vi "TestingPoint.vi"() -> ()   [LabVIEW 2016]
uses:
  <vilib>/Rock Robotics/WPI/Utilities/WPI_GetSetVariantRefNum.vi
panel:
  in  "Zero Yaw":bool
  in  "Config":T1={"Angle"=360.0, "MaxVelocity"=60.0, "MaxAccel"=50.0, "InitialVelocity"=0.0, "FinalVelocity"=0.0}
  out "Outputs":dbl(graph)
  in  "Go":bool
  in  "Go Backwards":bool
  out "Angular velocity":cluster{dbl, "vel":dbl}(graph)
  out "Angle":cluster{dbl, "pos":dbl}(graph)={50.0, "pos"=48.31556625}
  in  "Angular Constants":T2={"FF"=0.0066, "AFF"=0.0, "PID gains"={"P"=0.0, "I"=0.0, "D"=0.0}} {"PID gains"."D" format="%.3f"; "PID gains"."I" format="%.3f"; "PID gains"."P" format="%.3f"}
  # "MAKE DEFAULT"
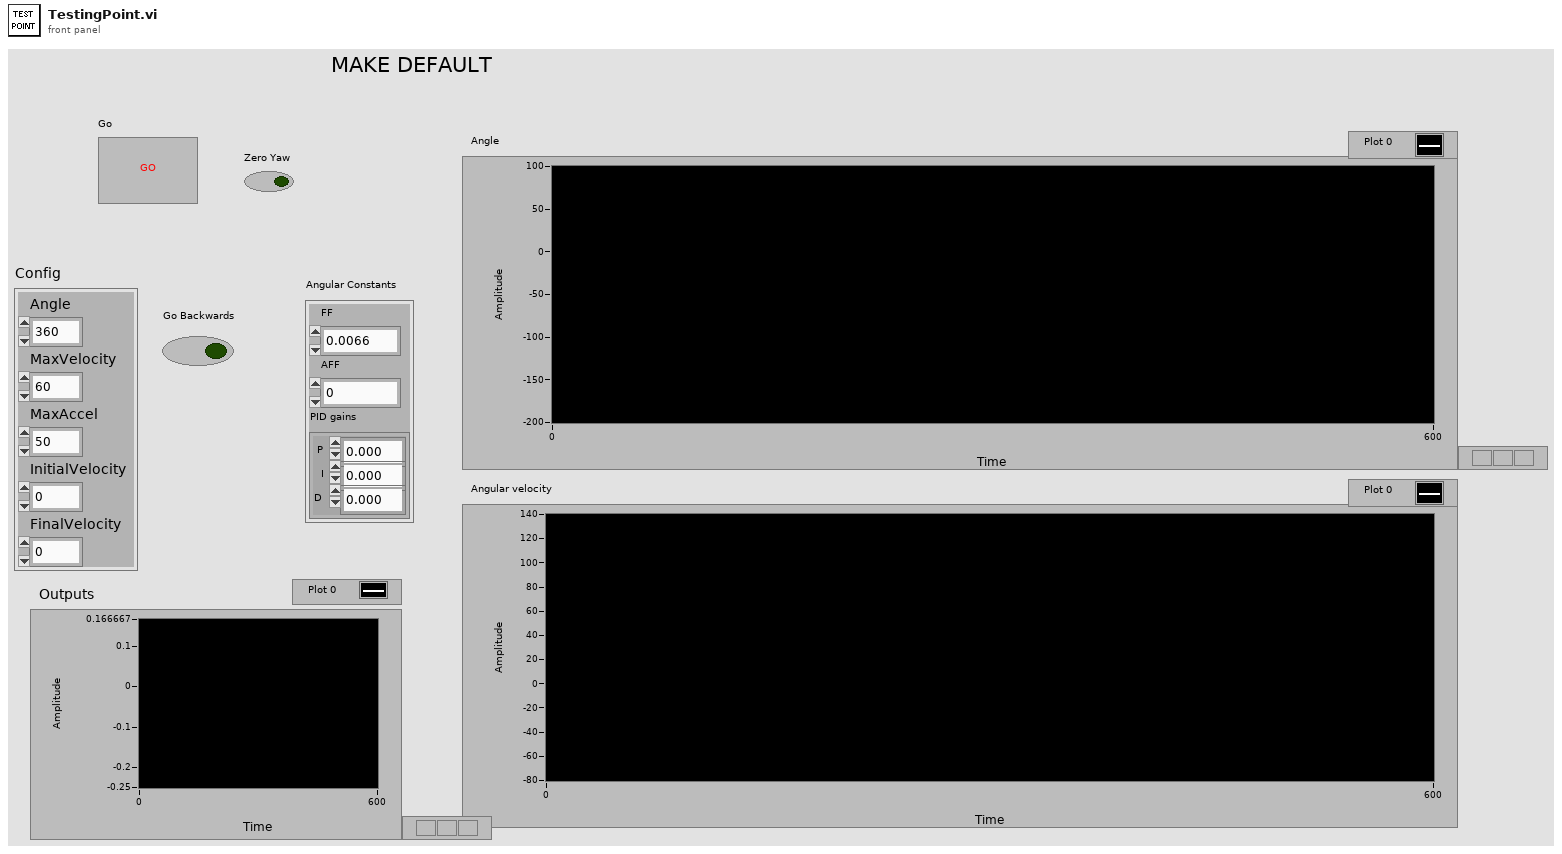
[diagram p1: front panel]
types:
  T1 = cluster{"Angle":dbl, "MaxVelocity":dbl, "MaxAccel":dbl, "InitialVelocity":dbl, "FinalVelocity":dbl}
  T2 = cluster{"FF":dbl, "AFF":dbl, "PID gains":cluster{"P":dbl, "I":dbl, "D":dbl}}
  T3 = cluster{"Yaw":dbl, "Roll":dbl, "Pitch":dbl, "Heading":dbl, "Fused Heading":dbl}
  T4 = typedef "WPI_RobotDriveDevRef.ctl" = cluster{"DevStatus":errorcluster, "Motors[]":T5[], "Square Inputs":bool, "Max Output":dbl}
  T5 = typedef "WPI_MotorControlDeviceRef.ctl" = cluster{"DeviceStatus":errorcluster, "Type":T6, "PWM":cluster{"PWM Channel":T7, "DeadBand":T8}, "CAN":cluster{"Device Number":u8, "SetOutput VI Ref":variant, "GetOutput VI Ref":variant, "Enable VI Ref":variant, "Disable VI Ref":variant, "Data":variant}, "Invert":bool}
  T6 = typedef "WPI_MotorControlType.ctl" = enum16{"PWM", "CAN"}
  T7 = typedef "FPGA_DIOPWMChannel.ctl" = enum8{"PWM 0", "PWM 1", "PWM 2", "PWM 3", "PWM 4", "PWM 5", "PWM 6", "PWM 7", "PWM 8", "PWM 9", "PWM MXP 0", "PWM MXP 1", "PWM MXP 2", "PWM MXP 3", "PWM MXP 4", "PWM MXP 5", "PWM MXP 6", "PWM MXP 7", "PWM MXP 8", "PWM MXP 9", "Invalid"}
  T8 = typedef "WPI_PWMDeadband.ctl" = cluster{"Name":string, "maxPositivePwm":i32, "minPositivePwm":i32, "centerPwm":i32, "maxNegativePwm":i32, "minNegativePwm":i32, "angularRange":u16}
  T9 = cluster{dbl, "distance/rotation":dbl, "distance/rotation":dbl}
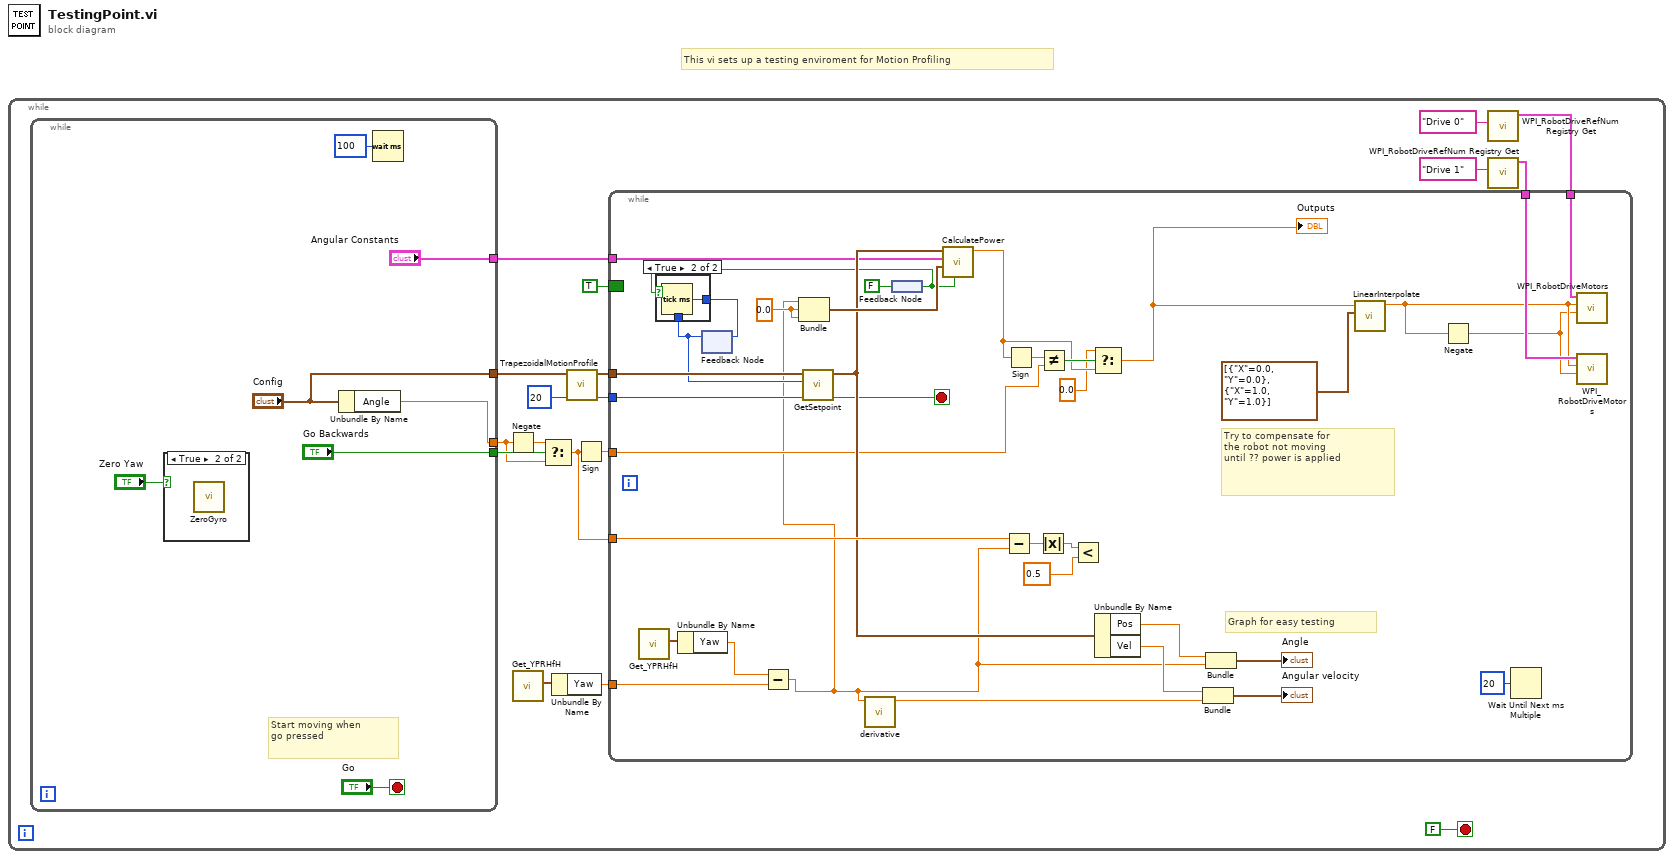
[diagram p0: block diagram]
diagram:
  # "This vi sets up a testing enviroment for Motion Profiling"
  n1 = while {
    stop <- FALSE stop-if-true
    n2 = while {
      tunnel: ["Go Backwards"] -> w8
      tunnel: [w22] -> w7
      tunnel: ["Config"] -> w6
      tunnel: ["Angular Constants"] -> w5
      stop <- "Go" stop-if-true
      # "Start moving when\ngo pressed"
      n3 = case shown="True" "Zero Yaw" {
        frame False {
        }
        frame True {
          n4 = call "ZeroGyro.vi"() -> ()  [unwired: 11 in, 1 out]
        }
      }
      n5 = Unbundle By Name("Config") -> ("Angle"=w22:dbl)
      n6 = Wait (ms)(milliseconds to wait=u32 100 ("millisecond multiple")) -> ()  [unwired: 1 out]
    }
    n7 = Negate(x=w7) -> (-x=w17:dbl)
    n8 = call <vilib>:"Get_YPRHfH.vi"() -> ("YRPHfH"=w2:T3)  [unwired: 11 in]
    n9 = Select(t=w17, s=w8, f=w7) -> (s? t:f=w10:dbl)
    n10 = Unbundle By Name(w2) -> ("Yaw"=w1:dbl)
    n11 = call "TrapezoidalMotionProfile.vi"("dt"=u32 20, "Config"=w6) -> ("dt"=w13:u32, "Profile"=w18:cluster{"Pos":dbl, "Vel":dbl, "Accel":dbl}[])  [unwired: 8 in]
    n12 = Sign(1:w10) -> (0:w9:dbl)
    n13 = call <vilib>:"WPI_RobotDriveRefNum Registry Get.vi"("refnum name"="Drive 0") -> ("RobotDriveDevRef"=w4:T4)  [unwired: 9 in, 1 out]
    n14 = call <vilib>:"WPI_RobotDriveRefNum Registry Get.vi"("refnum name"="Drive 1") -> ("RobotDriveDevRef"=w3:T4)  [unwired: 9 in, 1 out]
    n15 = while {
      tunnel: w18 -> [w52]
      tunnel: w10 -> [w57]
      border: TRUE ("Reset") -> [_]
      tunnel: w13 -> [w51]
      tunnel: w9 -> [w43]
      tunnel: w5 -> [w39]
      tunnel: w4 -> [w36]
      tunnel: w3 -> [w35]
      tunnel: w1 -> [w30]
      stop <- w45 stop-if-true
      w54 = 0.0 ("distance/rotation")
      # "Try to compensate for\nthe robot not moving\nuntil ?? power is applied"
      # "Graph for easy testing"
      n16 = call <vilib>:"Get_YPRHfH.vi"() -> ("YRPHfH"=w32:T3)  [unwired: 11 in]
      n17 = Unbundle By Name(w32) -> ("Yaw"=w31:dbl)
      n18 = feedback #1() -> (w37:u32)  [unwired: 1 in]
      n19 = Subtract(x=w31, y=w30) -> (x-y=w26:dbl)
      n20 = Bundle(w26, "distance/rotation"=w54, "distance/rotation"=w54) -> (w55:T9)  [unwired: 1 in]
      n21 = call "GetSetpoint.vi"("dt"=w51, "Start Time"=w37, "Profile"=w52) -> ("Profile done?"=w45:bool, "Setpoints"=w50:cluster{"Pos":dbl, "Vel":dbl, "Accel":dbl})  [unwired: 7 in]
      n22 = call "derivative.vi"("x"=w26) -> ("dx/dt"=w56:dbl)  [unwired: 10 in]
      n23 = feedback-in #2(FALSE ("Reset")) -> ()
      n24 = feedback #2() -> (w33:bool)
      n25 = case shown="True" w33 {
        tunnel: [w62 w63] -> w38
        tunnel: w37 -> [w62 _]
        frame False {
        }
        frame True {
          n26 = Tick Count (ms)() -> (millisecond timer value=w63:u32)
        }
      }
      n27 = feedback-in #1(w38) -> ()
      n28 = call "CalculatePower.vi"("Reset"=w33, "Process Variables"=w55, "Constants"=w39, "Setpoints"=w50) -> ("Power"=w41:dbl)  [unwired: 7 in]
      n29 = Subtract(x=w57, y=w26) -> (x-y=w60:dbl)
      n30 = Sign(1:w41) -> (0:w44:dbl)
      n31 = Absolute Value(x=w60) -> (abs(x)=w59:dbl)
      n32 = Not Equal?(x=w44, y=w43) -> (x != y?=w42:bool)
      n33 = Less?(x=w59, y=0.5 ("Closeness at end")) -> ()  [unwired: 1 out]
      n34 = Select(t=0.0, s=w42, f=w41) -> (s? t:f=w29:dbl)
      "Outputs" <- w29
      n35 = Unbundle By Name(w50) -> ("Pos"=w49:dbl, "Vel"=w48:dbl)
      n36 = Bundle("Vel"=w48, "dx/dt"=w56) -> (→"Angular velocity":cluster{"Vel":dbl, "dx/dt":dbl})  [unwired: 1 in]
      n37 = Bundle("Pos"=w49, w26) -> (→"Angle":cluster{"Pos":dbl, dbl})  [unwired: 1 in]
      n38 = call "LinearInterpolate.vi"("Points"=cluster{"X":dbl, "Y":dbl}[] [{"X"=0.0, "Y"=0.0}, {"X"=1.0, "Y"=1.0}], "Value"=w29) -> ("Output"=w28:dbl)  [unwired: 9 in]
      n39 = Negate(x=w28) -> (-x=w27:dbl)
      n40 = Wait Until Next ms Multiple(millisecond multiple=u32 20) -> ()  [unwired: 1 out]
      n41 = call <vilib>:"WPI_RobotDriveMotors.vi"("RightSpeed"=w27, "LeftSpeed"=w28, "RobotDriveDevRef"=w36) -> ()  [unwired: 6 in, 3 out]
      n42 = call <vilib>:"WPI_RobotDriveMotors.vi"("RightSpeed"=w27, "LeftSpeed"=w28, "RobotDriveDevRef"=w35) -> ()  [unwired: 6 in, 3 out]
    }
  }
